vi "Funnel_Execute.vi"   [LabVIEW 2020]
uses:
  Control_States_Funnel.ctl
  Funnel_Cluster.ctl
  Globals/Funnel_global.vi
types:
  T1 = typedef "Funnel_Cluster.ctl" = cluster{"Control States":T2, "Throttle":dbl}
  T2 = typedef "Control_States_Funnel.ctl" = enum16{"No_Op", "Manual_Op"}
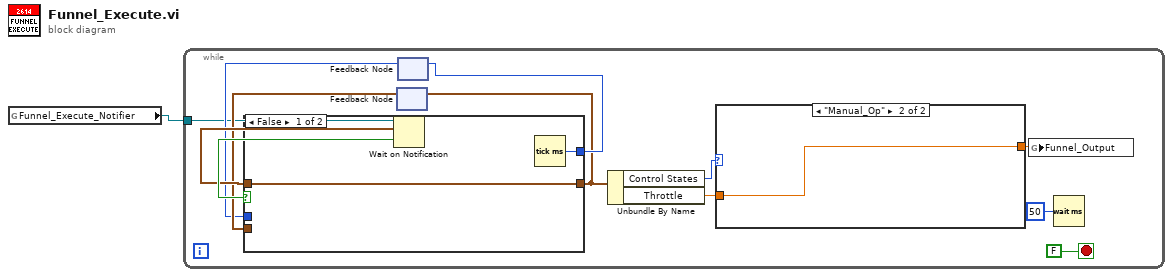
[diagram p0: block diagram]
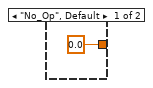
[diagram p2: hidden frame]
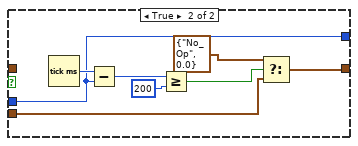
[diagram p3: hidden frame]
diagram:
  n1 = global read "Funnel_global.vi" "Funnel_Execute_Notifier"() -> (w1:refnum<notifier>)
  n2 = while {
    tunnel: w1 -> [w6]
    stop <- FALSE stop-if-true
    n3 = Wait on Notification(notifier=w6) -> (notification=w10:T1, timed out?=w11:bool)  [unwired: 3 in, 2 out]
    n4 = feedback #1() -> (w9:T1)  [unwired: 1 in]
    n5 = feedback #2() -> (w7:u32)  [unwired: 1 in]
    n6 = case shown="False" w11 {
      tunnel: w10 -> [w16 _]
      tunnel: [w16 w25] -> w5
      tunnel: w9 -> [_ w24]
      tunnel: [w17 w22] -> w8
      tunnel: w7 -> [_ w22]
      frame False {
        n7 = Tick Count (ms)() -> (millisecond timer value=w17:u32)
      }
      frame True {
        n8 = Tick Count (ms)() -> (millisecond timer value=w23:u32)
        n9 = Subtract(x=w23, y=w22) -> (x-y=w20:u32)
        n10 = Greater Or Equal?(x=w20, y=u32 200) -> (x >= y?=w21:bool)
        n11 = Select(t=T1 {"Control States"=enum."No_Op", "Throttle"=0.0} ("Funnel_Cluster"), s=w21, f=w24) -> (s? t:f=w25:T1)
      }
    }
    n12 = feedback-in #1(w5) -> ()
    n13 = feedback-in #2(w8) -> ()
    n14 = Unbundle By Name(w5) -> ("Control States"=w4:T2, "Throttle"=w2:dbl)
    n15 = case shown="\"Manual_Op\"" w4 {
      tunnel: [0.0 ("Funnel_Output") w15] -> w3
      tunnel: w2 -> [_ w15]
      frame "No_Op", Default {
      }
      frame "Manual_Op" {
      }
    }
    n16 = global write "Funnel_global.vi" "Funnel_Output"(w3) -> ()
    n17 = Wait (ms)(milliseconds to wait=u32 50) -> ()  [unwired: 1 out]
  }
